vi "RenderText_Blended.vi"(8 "No Error":errorcluster, 9 "FG Color":u32, 10 "Text":string, 11 "Font [TTF_Font *]":i64 format="%.0x") -> (0 "error out":errorcluster, 3 "Surface [SDL_Surface *]":i64 format="%.0x")   [LabVIEW 2026, in "SDL3.lvlib" / "TTF.lvlib"]
doc: "<B>Summary</B>\nRender UTF-8 text at high quality to a new ARGB surface.\n\n<B>Remarks</B>\nThis function will allocate a new 32-bit, ARGB surface, using alpha blending to dither the font with the given color. This function returns the new surface, or NULL if there was an error.\n\nThis will not word-wrap the string; you'll get a surface with a single line of text, as long as the string requires. You can use <B>TTF_RenderText_Blended_Wrapped()</B> instead if you need to wrap the output to multiple lines.\n\nThis will not wrap on newline characters.\n\nYou can render at other quality levels with <B>TTF_RenderText_Solid</B>, <B>TTF_RenderText_Shaded</B>, and <B>TTF_RenderText_LCD</B>."
uses:
  TTF.lvlib
  <vilib>/Utility/error.llb/Error Cluster From Error Code.vi
  Error/Error.lvlib
  Lib/SDL3_ttf.dll
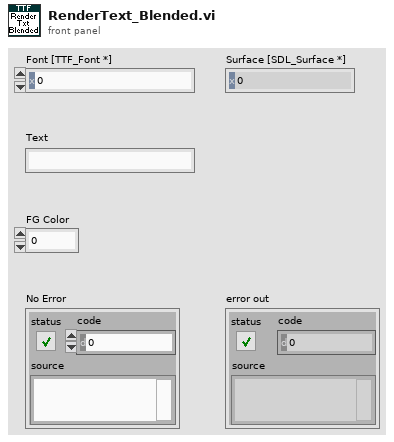
[diagram p1: front panel]
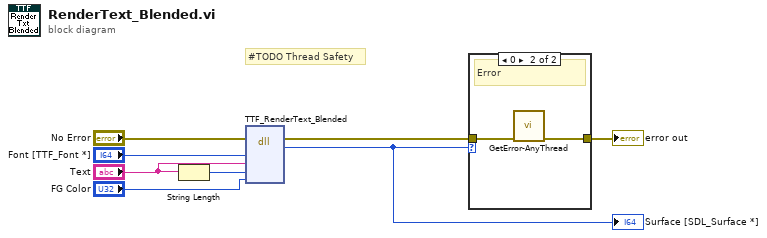
[diagram p0: block diagram]
diagram:
  # "#TODO Thread Safety"
  n1 = String Length(string="Text") -> (length=w3:i32)
  n2 = dll-call lib="C:/Users/saukko/Dev/LV-SDL3/Sources/SDL3/Lib/SDL3_ttf.*" fn="TTF_RenderText_Blended"(error in="No Error", "font"="Font [TTF_Font *]", "text"="Text", "length"=w3, "fg"="FG Color") -> (error out=w6:errorcluster, "return type"=w1:i64)  [unwired: 6 in, 1 out]
  "Surface [SDL_Surface *]" <- w1
  n3 = case shown="0" w1 {
    tunnel: w6 -> [w9 w11]
    tunnel: [w9 w10] -> w7
    frame Default {
      # "Ok"
    }
    frame 0 {
      # "Error"
      n4 = call "GetError-AnyThread.vi"("No Error"=w11) -> ("Error Out"=w10:errorcluster)  [unwired: 10 in]
    }
  }
  "error out" <- w7
